vi "SVX Orbit and Timebase Plot (Filtered) (N Ch - 1 Order).vi"(0 "magnitudes [RMS]":T1(array[cluster]) {"magnitude" format="%.2f"; "time/rev/RPM" format="%.2f"}, 1 "samples/rev wanted":i32=64, 2 "reset? (F)":bool, 5 "phases [phase lag]":cluster{"time/rev/RPM":dbl[], "phase":dbl[]}[](array[cluster]) {"phase" format="%.2f"; "time/rev/RPM" format="%.2f"}, 7 "magnitude/phase position info":T10, 9 "magnitudes info":T3[](array[typedef]) {"x-axis units" items=["Time (s)"=0, "Frequency-CB (Hz)"=1, "Frequency-CPB (Hz)"=1248, "Frequency-Arbitrary (Hz)"=2357, "Quefrency (s)"=2, "Revolutions (rev)"=3, "Order"=4, "Speed (RPM)"=11, "Speed (rad/s)"=21, "Index"=65535]; "weighting filter" items=["Linear", "A-weighting", "B-weighting", "C-weighting", "ITU-R 468-4", "Dolby", "CCITT", "C-message", "Wb", "Wc", "Wd", "We", "Wf", "Wh", "Wj", "Wk", "Wm", "AES17 20 kHz lowpass", "AES17 40 kHz lowpass", "AES17 20 kHz highpass", "AES17 40 kHz highpass"]; "dB reference [EU]" format="%.2f"; "engineering units" items=["custom..."=0, "V"=1, "A"=21, "C"=30, "pC"=31, "s"=32, "-"=29, "Pa"=2, "N"=20, "g"=3, "m/s^2"=4, "m/s"=5, "m"=6, "mm/s"=12, "mm"=13, "micron/s"=14, "micron"=15, "in/s^2"=7, "in/s"=8, "in"=9, "mil/s"=10, "mil"=11, "rad/s^2"=16, "rad/s"=17, "rad"=18, "deg/s^2"=26, "deg/s"=27, "deg"=28, "RPM"=22, "cycle/s^2"=23, "Hz"=24, "cycle"=25, "strain"=19]; "spectral info"."window" items=["None "=0, "Hanning"=1, "Hamming"=2, "Blackman-Harris"=3, "Exact Blackman"=4, "Blackman"=5, "Flat Top"=6, "4 Term B-Harris "=7, "7 Term B-Harris"=8, "Low Sidelobe"=9, "Force - Exponential"=10, "Gaussian"=62]}, 11 "error in (no error)":errorcluster, 12 "channel properties":T2[](array[typedef]) {"probe angle [deg]" max=360; "direction" items=["CCW", "CW"]}, 13 "segment settings":cluster{"start [rev]":dbl, "end [rev]":dbl}={"start [rev]"=0.0, "end [rev]"=inf}) -> (4 "orbit/timebase plot":T9(array[cluster]), 10 "end reached?":bool, 14 "actual segment settings":cluster{"start [rev]":dbl, "end [rev]":dbl}, 15 "error out":errorcluster)   [LabVIEW 2017, in "SoundVib_MCMDisplay.lvlib"]
doc: "Prepares unfiltered or filtered orbit plot data or timebase plot data for displaying on an Orbit Plot or Timebase Plot. Use this VI to prepare magnitude and phase data for entry into an orbit or timebase plot. Wire data to the <B>even-angle signals</B> input to determine the polymorphic instance to use or manually select the instance."
uses:
  <vilib>/addons/Sound and Vibration/Order Analysis/Data Presentation/SoundVib_MCMDisplay.lvlib
  <vilib>/addons/Sound and Vibration/Order Analysis/Misc/OAT Position Info.ctl
  <vilib>/addons/_NISVFA/_Shared subVIs/Controls/svc_Spectrum Info.ctl
  <vilib>/addons/_NISVFA/_Shared subVIs/Controls/svc_X-Axis Units.ctl
  <vilib>/addons/_NISVFA/_Shared subVIs/Controls/svc_Spectrum Type.ctl
  <vilib>/addons/_NISVFA/_Shared subVIs/Controls/svc_Engineering Units Text Ring.ctl
  <vilib>/addons/_NISVFA/_Shared subVIs/Controls/svc_Weighting Filter Text Ring.ctl
  <vilib>/addons/_NISVFA/_Shared subVIs/Controls/svc_Complimentary Spectrum Units.ctl
  <vilib>/addons/Sound and Vibration/Order Analysis/Data Presentation/SubVIs/OAT MCM Channel Property.ctl
  <vilib>/addons/Sound and Vibration/Order Analysis/Resample Order Tracking/SoundVib_Resampling.lvlib
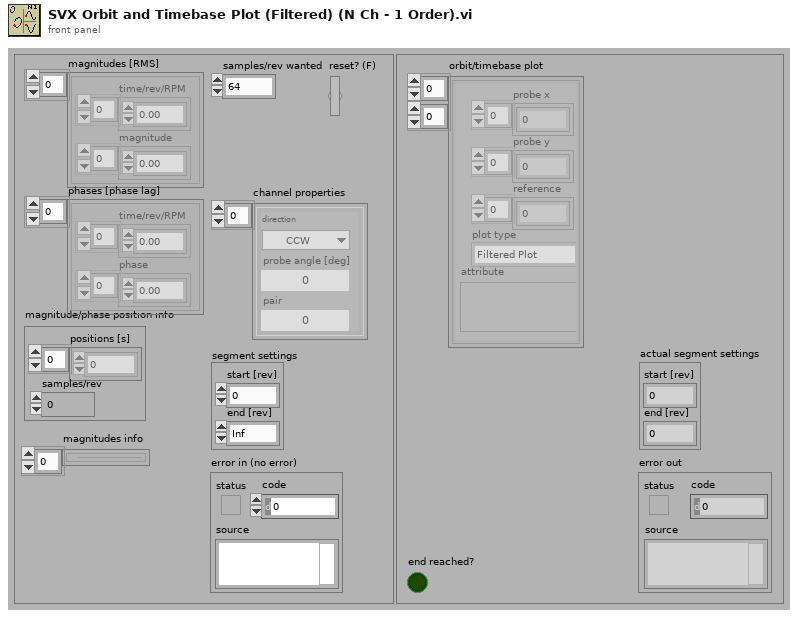
[diagram p1: front panel]
types:
  T1 = cluster{"time/rev/RPM":dbl[], "magnitude":dbl[]}[]
  T2 = typedef "OAT MCM Channel Property.ctl" = cluster{"direction":u16, "probe angle [deg]":u16, "pair":u16}
  T3 = typedef "svc_Spectrum Info.ctl" = cluster{"channel name":string, "description":string, "x-axis units":T4, "spectral info":cluster{"spectrum type":T5, "linear/dB":enum16{"linear", "dB"}, "window":u16, "window size":i32, "FFT size":i32}, "engineering units":T6, "custom label":string, "dB reference [EU]":dbl, "peak units":enum16{"rms", "peak", "peak-peak"}, "weighting filter":T7, "spectral density?":bool, "unit label":string, "spectrum skewed?":bool, "complimentary spectrum units":T8}
  T4 = typedef "svc_X-Axis Units.ctl" = u16
  T5 = typedef "svc_Spectrum Type.ctl" = enum16{"FFT Spectrum [complex]", "Amplitude [Magnitude]", "Power [Magnitude^2]", "Cross Spectrum [complex]", "Frequency Response [Complex]"}
  T6 = typedef "svc_Engineering Units Text Ring.ctl" = u16
  T7 = typedef "svc_Weighting Filter Text Ring.ctl" = u16
  T8 = typedef "svc_Complimentary Spectrum Units.ctl" = enum16{"none", "radians", "degrees", "cycles", "imaginary"}
  T9 = cluster{"probe x":dbl[], "probe y":dbl[], "reference":dbl[], "plot type":enum16{"Filtered Plot", "Unfiltered Plot"}, "attribute":variant}[][]
  T10 = typedef "OAT Position Info.ctl" = cluster{"positions [s]":dbl[], "samples/rev":dbl}
  T11 = cluster{"dB on? (F)":bool, "unwrap phase? (T)":bool, "unit in degree? (T)":bool}
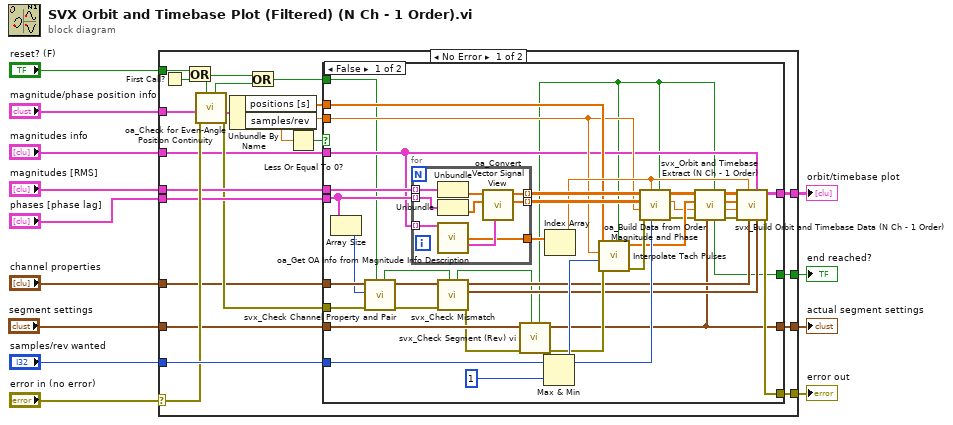
[diagram p0: block diagram]
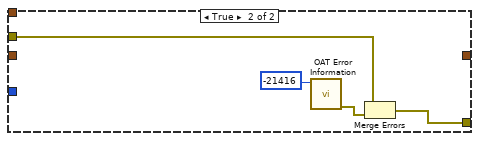
[diagram p2: hidden frame]
diagram:
  n1 = case shown="No Error" "error in (no error)" {
    selector: "error in (no error)" -> [w24 w88]
    tunnel: [w34 w88] -> w12
    tunnel: "samples/rev wanted" -> [w35 _]
    tunnel: "magnitude/phase position info" -> [w29 _]
    tunnel: "reset? (F)" -> [w31 _]
    tunnel: [w23 _] -> w4
    tunnel: "magnitudes [RMS]" -> [w22 _]
    tunnel: "phases [phase lag]" -> [w21 _]
    tunnel: "magnitudes info" -> [w19 _]
    tunnel: "channel properties" -> [w18 _]
    tunnel: "segment settings" -> [w16 _]
    tunnel: [w15 _] -> w2
    tunnel: [w14 _] -> w1
    frame No Error {
      n2 = First Call?() -> (First Call?: T/F=w30:bool)
      n3 = Or(x=w31, y=w30) -> (x .or. y?=w28:bool)
      n4 = call <vilib>:"oa_Check for Even-Angle Position Continuity.vi"("reset in"=w28, "error in (no error)"=w24, "even-angle position info"=w29) -> ("error out"=w20:errorcluster, "even-angle position info dup"=w25:T10, "position not continuous"=w27:bool)  [unwired: 6 in]
      n5 = Unbundle By Name(w25) -> ("positions [s]"=w17:dbl[], "samples/rev"=w32:dbl)
      n6 = Or(x=w28, y=w27) -> (x .or. y?=w26:bool)
      n7 = Less Or Equal To 0?(x=w32) -> (x <= 0?=w33:bool)
      n8 = case shown="False" w33 {
        tunnel: w35 -> [w74 _]
        tunnel: [w65 w85] -> w34
        tunnel: w32 -> [w61 _]
        tunnel: w26 -> [w53 _]
        tunnel: [w66 _] -> w23
        tunnel: w22 -> [w70 _]
        tunnel: w21 -> [w68 _]
        tunnel: w20 -> [w69 w84]
        tunnel: w19 -> [w57 _]
        tunnel: w18 -> [w67 _]
        tunnel: w17 -> [w62 _]
        tunnel: w16 -> [w59 _]
        tunnel: [w41 _] -> w15
        tunnel: [w36 _] -> w14
        frame False {
          n9 = Array Size(array=w68) -> (size(s)=w56:i32)
          n10 = call <vilib>:"svx_Check Channel Property and Pair.vi"("reset in"=w53, "error in (no error)"=w69, "channel number"=w56, "channel property"=w67) -> ("error out"=w55:errorcluster, "channel property out"=w54:T2[], "reset out"=w52:bool)  [unwired: 5 in]
          n11 = for {
            tunnel: w70 -> [w83] mode=indexing
            tunnel: w68 -> [w82] mode=indexing
            tunnel: [w79] -> w72 mode=indexing
            tunnel: [w78] -> w71 mode=indexing
            tunnel: w57 -> [w75] mode=indexing
            tunnel: [w76] -> w64
            n12 = Unbundle(w83) -> ("magnitude"=w81:dbl[])  [unwired: 1 out]
            n13 = Unbundle(w82) -> ("phase"=w80:dbl[])  [unwired: 1 out]
            n14 = call <vilib>:"oa_Get OA Info from Magnitude Info Description.vi"("magnitude info"=w75) -> ("orders to compute"=w76:dbl[], "view"=w77:T11)  [unwired: 10 in, 3 out]
            n15 = call <vilib>:"oa_Convert Vector Signal View.vi"("view"=w77, "phase"=w80, "magnitude"=w81) -> ("phase out"=w78:dbl[], "magnitude out"=w79:dbl[])  [unwired: 7 in]
          }
          n16 = call <vilib>:"svx_Check Mismatch.vi"("reset in"=w52, "error in (no error)"=w55, "channel property in"=w54) -> ("error out"=w51:errorcluster, "pair index"=w49:cluster{"index 1":i32, "index 2":i32}[], "channel property out"=w50:T2[], "reset out"=w48:bool)  [unwired: 5 in]
          n17 = call <vilib>:"svx_Check Segment (Rev) vi.vi"("reset in"=w48, "error in (no error)"=w51, "segment settings"=w59) -> ("error out"=w58:errorcluster, "actual segment settings"=w41:cluster{"start [rev]":dbl, "end [rev]":dbl}, "reset out"=w42:bool)  [unwired: 6 in]
          n18 = Max & Min(x=w74, y=1 ("x")) -> (max(x,y)=w60:i32)  [unwired: 1 out]
          n19 = Index Array(array=w64) -> (element=w63:dbl)  [unwired: 1 in]
          n20 = call <vilib>:"Interpolate Tach Pulses.vi"("reset? (True)"=w42, "error in (no error)"=w58, "pulse/revolution wanted"=w60, "pulse/revolution (1)"=w61, "pulse positions [s]"=w62) -> ("error out"=w47:errorcluster, "interpolated pulse positions[s]"=w45:dbl[])  [unwired: 4 in, 1 out]
          n21 = call <vilib>:"oa_Build Data from Order Magnitude and Phase.vi"("reset? (F)"=w42, "samples/revolution wanted"=w60, "order"=w63, "error in (no error)"=w47, "samples/revolution"=w61, "phase lag"=w71, "magnitude"=w72) -> ("error out"=w43:errorcluster, "actual samples/rev"=w44:dbl, "order waveform"=w46:dbl[][])  [unwired: 2 in]
          n22 = call <vilib>:"svx_Orbit and Timebase Extract (N Ch - 1 Order).vi"("reset? (F)"=w42, "segment settings"=w41, "error in (no error)"=w43, "actual samples/rev in"=w44, "interpolated pulse positions in"=w45, "order data in"=w46) -> ("error out"=w37:errorcluster, "actual samples/rev out"=w38:dbl, "interpolated pulse positions out"=w39:dbl[], "order data out"=w40:dbl[][], "end reached"=w36:bool)  [unwired: 1 in]
          n23 = call <vilib>:"svx_Build Orbit and Timebase Data (N Ch - 1 Order).vi"("pair index"=w49, "magnitudes info"=w57, "channel properties"=w50, "order"=w63, "error in (no error)"=w37, "actual samples/rev"=w38, "interpolated pulse positions[s]"=w39, "order data"=w40) -> ("error out"=w65:errorcluster, "orbit/timebase plot"=w66:T9)  [unwired: 2 in]
        }
        frame True {
          n24 = call <vilib>:"OAT Error Information.vi"("error code"=-21416) -> ("error out"=w86:errorcluster)  [unwired: 6 in]
          n25 = Merge Errors(w84, w86) -> (w85:errorcluster)
        }
      }
    }
    frame Error {
    }
  }
  "error out" <- w12
  "orbit/timebase plot" <- w4
  "end reached?" <- w1
  "actual segment settings" <- w2
